vi "SetBufferCollectTimestamps.vi"(7 "SMU":T1, 8 "Error In":errorcluster, 9 "Enable?":bool, 10 "Buffer":u8=1 min=1 max=2 step=1, 11 "Keithley 2602 In":refnum<visa-resource-name>) -> (0 "Error Out":errorcluster, 3 "Keithley 2602 Out":refnum<visa-resource-name>)   [LabVIEW 2012, in "Keithley-2602.lvlib"]
uses:
  Keithley-2602.lvlib
  Controls/SMU.ctl
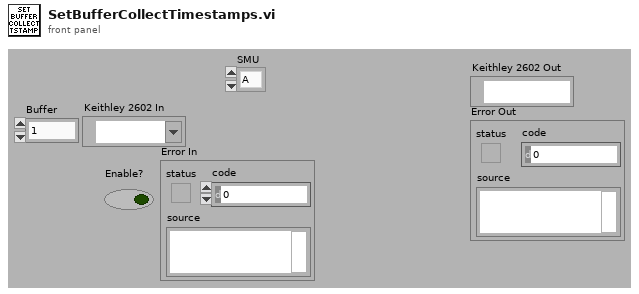
[diagram p1: front panel]
types:
  T1 = typedef "Keithley-2602.lvlib/SMU.ctl" = enum16{"A", "B"}
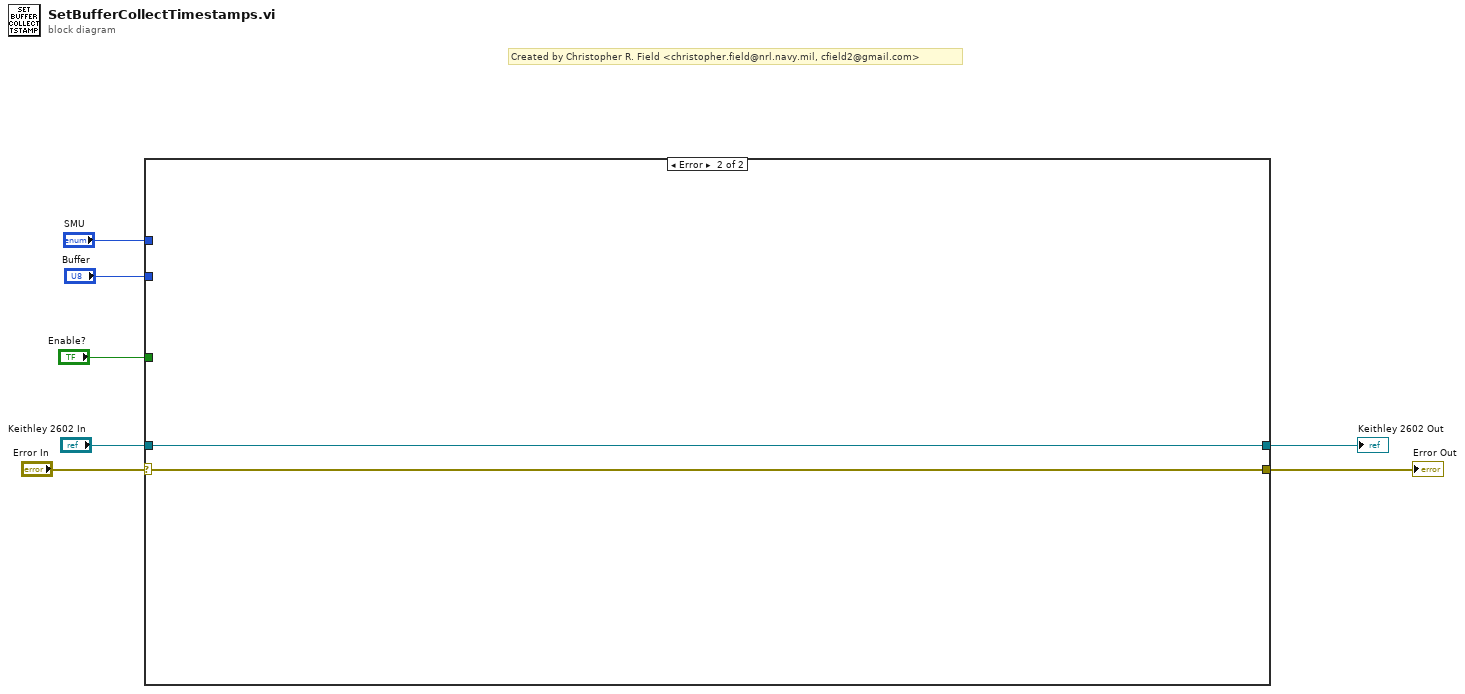
[diagram p0: block diagram]
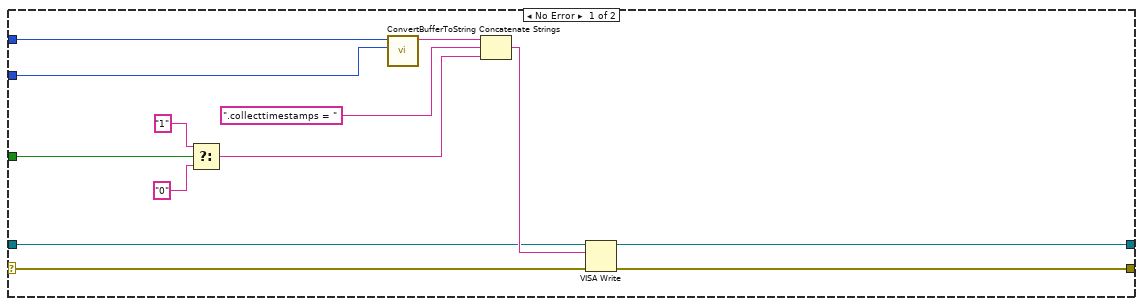
[diagram p2: hidden frame]
diagram:
  # "Created by Christopher R. Field <christopher.field@nrl.navy.mil, cfield2@gmail.com>"
  n1 = case shown="Error" "Error In" {
    selector: "Error In" -> [w8 w21]
    tunnel: "Buffer" -> [w20 _]
    tunnel: "Enable?" -> [w19 _]
    tunnel: "Keithley 2602 In" -> [w12 w22]
    tunnel: [w11 w22] -> w4
    tunnel: [w10 w21] -> w3
    tunnel: "SMU" -> [w9 _]
    frame No Error {
      n2 = Select(t="1", s=w19, f="0") -> (s? t:f=w14:string)
      n3 = call "ConvertBufferToString.vi"("Buffer"=w20, "SMU"=w9) -> ("Buffer"=w16:string)  [unwired: 9 in]
      n4 = Concatenate Strings(w16, ".collecttimestamps = ", w14) -> (w13:string)
      n5 = VISA Write(VISA resource name=w12, write buffer=w13, error in (no error)=w8) -> (VISA resource name out=w11:refnum<visa-resource-name>, error out=w10:errorcluster)  [unwired: 1 out]
    }
    frame Error {
    }
  }
  "Keithley 2602 Out" <- w4
  "Error Out" <- w3
